vi "HRR-trataArquivo.vi"(8 "error in (no error)":errorcluster, 10 "arquivo na home":path, 11 "arquivo no U":path) -> (0 "error out":errorcluster)   [LabVIEW 2019]
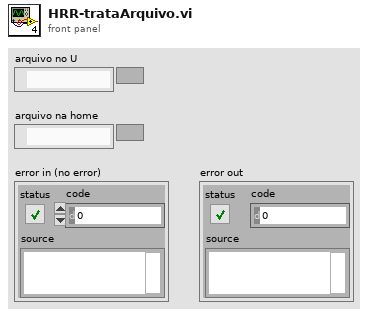
[diagram p1: front panel]
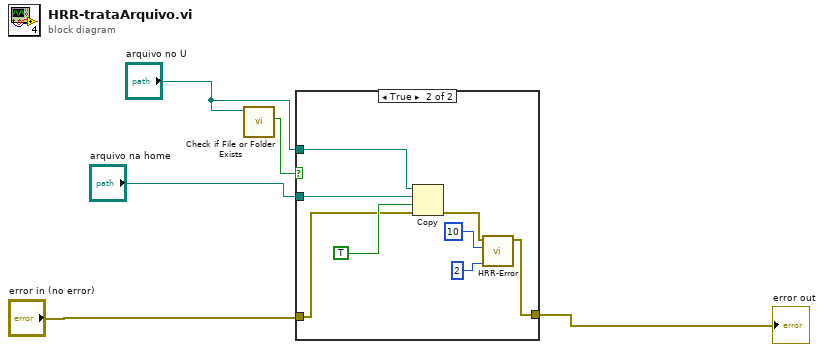
[diagram p0: block diagram]
diagram:
  n1 = call <vilib>:"Check if File or Folder Exists.vi"("path"="arquivo no U") -> ("file or folder exists?"=w3:bool)  [unwired: 8 in, 2 out]
  n2 = case shown="True" w3 {
    tunnel: [w6 w10] -> w2
    tunnel: "error in (no error)" -> [w6 w9]
    tunnel: "arquivo no U" -> [_ w8]
    tunnel: "arquivo na home" -> [_ w7]
    frame False {
    }
    frame True {
      n3 = Copy(8:w9, 9:TRUE ("overwrite (F)"), 10:w7, 11:w8) -> (0:w11:errorcluster)  [unwired: 1 in, 2 out]
      n4 = call "HRR-Error.vi"("Status"=u8 2, "Nvezes"=10, "error in (no error)"=w11) -> ("error out"=w10:errorcluster)  [unwired: 8 in]
    }
  }
  "error out" <- w2
